vi "On-Off Epoxy.vi"   [LabVIEW 2016]
uses:
  Classes/Controller/Dispenser/Dispenser.lvclass
  Classes/Controller/Controller.lvclass
types:
  T1 = typedef "Controller.lvclass/Controllers.ctl" = cluster{"I-O.lvclass":refnum<class "I-O.lvclass">, "Motion.lvclass":refnum<class "Motion.lvclass">, "Dispenser.lvclass":refnum<class "Dispenser.lvclass">}
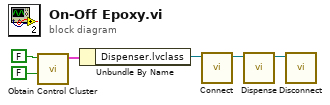
[diagram p0: block diagram]
diagram:
  n1 = call "Obtain Control Cluster.vi"("I/O"=FALSE, "Motion"=FALSE) -> ("Control Out"=w4:T1)  [unwired: 9 in]
  n2 = Unbundle By Name(w4) -> ("Dispenser.lvclass"=w3:refnum<class "Dispenser.lvclass">)
  n3 = call-dynamic "Connect.vi"("Controller in"=w3) -> ("Controller out"=w6:refnum<class "Dispenser.lvclass">)  [unwired: 9 in, 1 out]
  n4 = call-dynamic "Dispense.vi"("Dispenser in"=w6) -> ("Dispenser out"=w5:refnum<class "Dispenser.lvclass">)  [unwired: 9 in, 1 out]
  n5 = call-dynamic "Disconnect.vi"("Controller in"=w5) -> ()  [unwired: 9 in, 1 out]
